vi "LtaSet.vi"(8 "Error In":errorcluster[](array[cluster]), 10 "Data":variant) -> (0 "Error Out":errorcluster[](array[cluster]), 2 "BusNum":i32)   [LabVIEW 2017, in "Bus_class.lvlib" / "Bus.lvclass"]
uses:
  Bus.lvclass
  TestAutomation/Comms/CommsData.ctl
  <vilib>/Utility/error.llb/Error Cluster From Error Code.vi
  <vilib>/ErrorRing/Error Ring.xnode
  TestAutomation/Comms/Comms.lvlib
  <userlib>/NIST/NISTErrorLib/NISTErrorLib.lvlib
  TestAutomation/LTA/LTA.lvlib
  Framework.lvlib
panel:
  out "XMLData":string
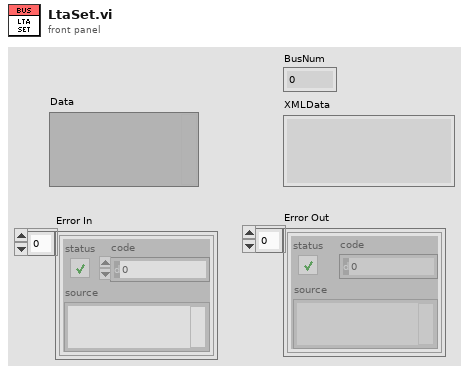
[diagram p1: front panel]
types:
  T1 = typedef "Comms.lvlib/CommsData.ctl" = cluster{"Command":string, "XMLData":string}
  T2 = typedef "Framework.lvlib/clFrameworkData.ctl" = cluster{"EvtINIFilePaths":path[], "BusClassInstances":refnum<class "Bus.lvclass">[], "PmuImpairINIFilePaths":path[], "FlagImpairINIFilePaths":path[], "NetImpairINIFilePaths":path[], "OutputToFileINIFilePaths":path[], "AppINIFilePaths":path[], "AppModuleID":i32, "OutputToFileID":i32}
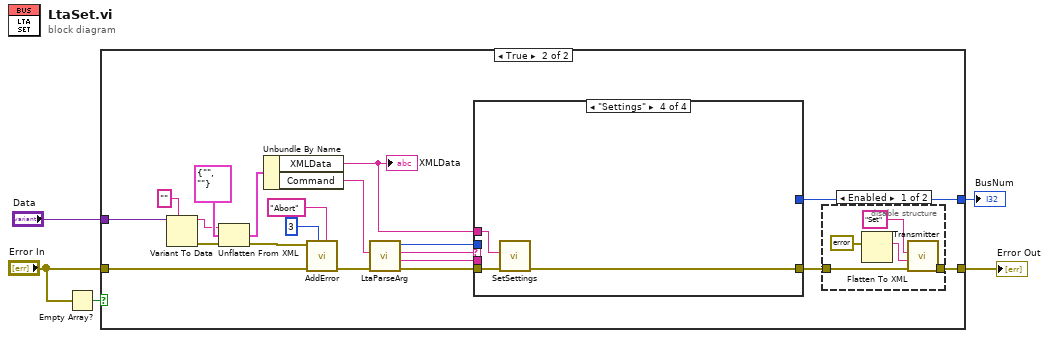
[diagram p0: block diagram]
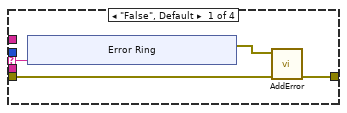
[diagram p4: hidden frame]
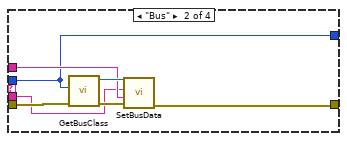
[diagram p5: hidden frame]
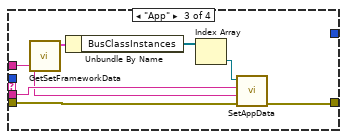
[diagram p6: hidden frame]
diagram:
  n1 = Empty Array?(array="Error In") -> (empty?=w5:bool)
  n2 = case shown="True" w5 {
    tunnel: "Error In" -> [w6 w18]
    tunnel: "Data" -> [_ w17]
    tunnel: [w6 w7] -> w2
    tunnel: [_ w9] -> w1
    frame False {
    }
    frame True {
      n3 = Variant To Data(type="", Variant=w17) -> (data=w21:string, error out=w20:errorcluster)  [unwired: 1 in]
      n4 = Unflatten From XML(xml string=w21, type=T1 {"Command"="", "XMLData"=""} ("CommsData"), error in (no error)=w20) -> (value=w26:T1, error out=w23:errorcluster)
      n5 = Unbundle By Name(w26) -> ("XMLData"=w10:string, "Command"=w13:string)
      "XMLData" <- w10
      n6 = call <userlib>:"AddError.vi"("Severity"="Abort", "Priority"=u8 3, "ErrorArray"=w18, "error in (no error)"=w23) -> ("ErrorArray"=w16:errorcluster[])  [unwired: 6 in, 1 out]
      n7 = call "LtaParseArg.vi"("Error In"=w16, "Arg In"=w13) -> ("Error Out"=w15:errorcluster[], "ArgRemaining"=w11:string, "Arg 1"=w12:string, "Arg1Num"=w14:i32)  [unwired: 6 in]
      n8 = case shown="\"Settings\"" w12 {
        selector: w12 -> [w36 _ _ _]
        tunnel: w15 -> [w34 w50 w54 w60]
        tunnel: w14 -> [_ w45 _ _]
        tunnel: w11 -> [_ w44 w57 _]
        tunnel: [w33 w46 w55 w59] -> w8
        tunnel: w10 -> [_ w47 w56 w58]
        tunnel: [_ w45 _ _] -> w9
        frame "False", Default {
          n9 = xnode "Error Ring"("parameter 0"=w36) -> ("error out"=w35:errorcluster)
          n10 = call <userlib>:"AddError.vi"("ErrorArray"=w34, "error in (no error)"=w35) -> ("ErrorArray"=w33:errorcluster[])  [unwired: 8 in, 1 out]
        }
        frame "Bus" {
          n11 = call "GetBusClass.vi"("ErrorArray In"=w50, "BusNumber"=w45) -> ("ErrorArray Out"=w49:errorcluster[], "Framework.lvlib:Bus.lvclass"=w48:refnum<class "Bus.lvclass">)  [unwired: 8 in]
          n12 = call "SetBusData.vi"("Error In"=w49, "XmlData"=w47, "arg"=w44, "Bus in"=w48) -> ("Error Out"=w46:errorcluster[])  [unwired: 6 in, 1 out]
        }
        frame "App" {
          n13 = call "GetSetFrameworkData.vi"() -> ("clFrameworkData Out"=w53:T2)  [unwired: 11 in]
          n14 = Unbundle By Name(w53) -> ("BusClassInstances"=w51:refnum<class "Bus.lvclass">[])
          n15 = Index Array(array=w51) -> (element=w52:refnum<class "Bus.lvclass">)  [unwired: 1 in]
          n16 = call "SetAppData.vi"("Error In"=w54, "XmlData"=w56, "arg"=w57, "Bus in"=w52) -> ("Error Out"=w55:errorcluster[])  [unwired: 6 in, 1 out]
        }
        frame "Settings" {
          n17 = call "SetSettings.vi"("Error In"=w60, "XmlData"=w58) -> ("Error Out"=w59:errorcluster[])  [unwired: 9 in]
        }
      }
      n18 = disable-structure shown="Enabled" {
        disable-tunnel: w8 -> [w31 w32]
        disable-tunnel: [w30 w32] -> w7
        frame Enabled {
          n19 = Flatten To XML(anything=errorcluster {"status"=FALSE, "code"=0, "source"=""} ("error constant")) -> (xml string=w27:string)
          n20 = call "Transmitter.vi"("ErrorArray"=w31, "XMLData"=w27, "Command"="Set") -> ("ErrorArray"=w30:errorcluster[])  [unwired: 7 in, 1 out]
        }
        frame Disabled {
        }
      }
    }
  }
  "Error Out" <- w2
  "BusNum" <- w1
